vi "Initialize.vi"(8 "error in (no error)":errorcluster, 10 "Memory Size":i32) -> (0 "error out":errorcluster, 3 "Virtual Memory Unit out":refnum<class "Virtual Memory Unit.lvclass">)   [LabVIEW 2020, in "BCI-1553 API.lvlib" / "Virtual Memory.lvlib" / "Virtual Memory Unit.lvclass"]
doc: "Creates a Virtual Memory object that has a predefined static size."
uses:
  Virtual Memory Unit.lvclass
  Virtual Memory Unit.lvclass/Virtual Memory Unit.ctl
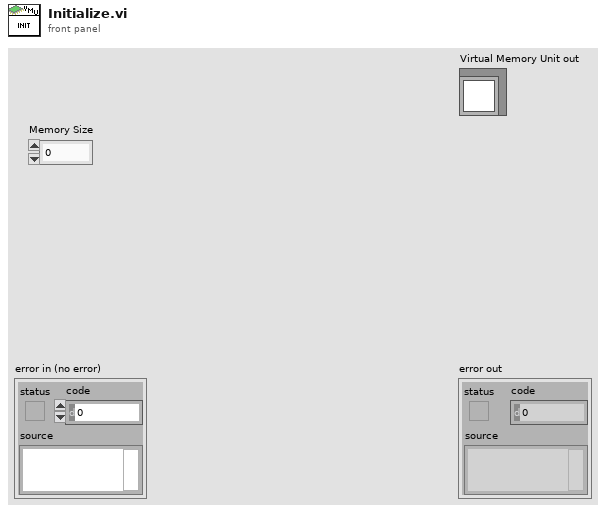
[diagram p1: front panel]
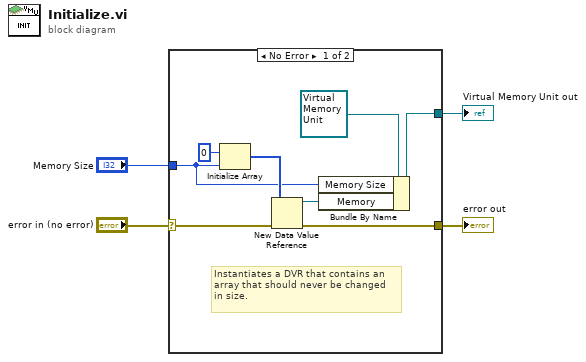
[diagram p0: block diagram]
diagram:
  n1 = case shown="No Error" "error in (no error)" {
    selector: "error in (no error)" -> [w9 w13]
    tunnel: [w10 w13] -> w3
    tunnel: [w6 _] -> w2
    tunnel: "Memory Size" -> [w5 _]
    frame No Error {
      # "Instantiates a DVR that contains an\narray that should never be changed\nin size."
      n2 = Initialize Array(u16 0, w5) -> (w11:u16[])
      n3 = New Data Value Reference(data value=w11, error in=w9) -> (data value reference=w8:refnum<data-value>, error out=w10:errorcluster)
      n4 = Bundle By Name(cluster=refnum<class "Virtual Memory Unit.lvclass"> refnum ("Virtual Memory Unit out"), "Memory Size"=w5, "Memory"=w8) -> (w6:refnum<class "Virtual Memory Unit.lvclass">)
    }
    frame Error {
    }
  }
  "error out" <- w3
  "Virtual Memory Unit out" <- w2
